vi "ArduinoCom.vi"(8 "error out":errorcluster, 10 "write buffer":string="b", 11 "VISA resource name out":refnum<visa-resource-name>) -> (0 "error out 2":errorcluster, 3 "VISA resource name out 2":refnum<visa-resource-name>)   [LabVIEW 2021]
panel:
  out "return count":u32=1
  out "Serial Settings:Number of Bytes at Serial Port":u32=3
  out "read buffer":string="a\r\n"
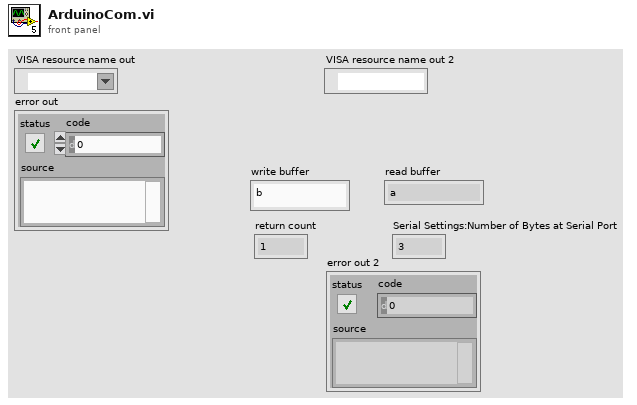
[diagram p1: front panel]
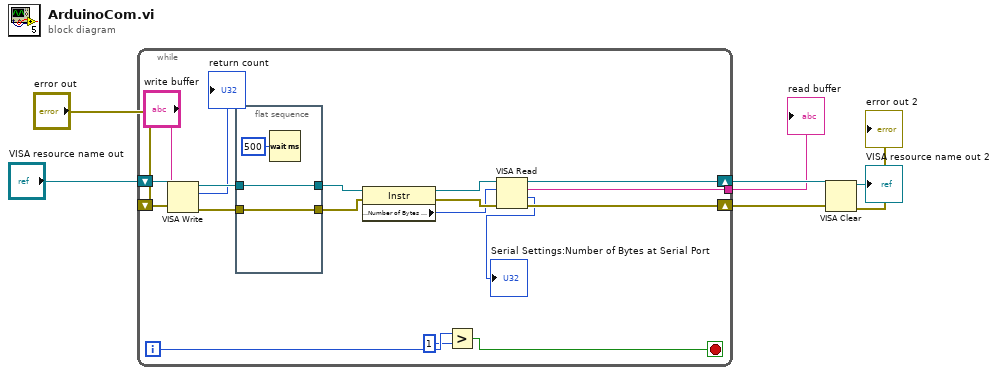
[diagram p0: block diagram]
diagram:
  n1 = while {
    tunnel: [w18] -> w5
    shift-right: [w19] -> w6
    shift-left: "error out" -> [w25]
    shift-right: [w20] -> w7
    shift-left: "VISA resource name out" -> [w24]
    i -> [w10]
    stop <- w8 stop-if-true
    n2 = VISA Write(VISA resource name=w24, write buffer="write buffer", error in (no error)=w25) -> (VISA resource name out=w22:refnum<visa-resource-name>, return count=→"return count":u32, error out=w21:errorcluster)
    n3 = flat-sequence {
      tunnel: w22 -> [w28]
      tunnel: [w28] -> w17
      tunnel: w21 -> [w27]
      tunnel: [w27] -> w16
      frame #0 {
        n4 = Wait (ms)(milliseconds to wait=u32 500) -> ()  [unwired: 1 out]
      }
    }
    n5 = property class="Instr"(reference=w17, error in=w16) -> (reference out=w15:refnum<visa-resource-name>, error out=w14:errorcluster, "Serial Settings:Number of Bytes at Serial Port"=w13:u32)
    n6 = Greater?(x=w10, y=1) -> (0:w8:bool)
    n7 = VISA Read(VISA resource name=w15, byte count=w13, error in (no error)=w14) -> (VISA resource name out=w20:refnum<visa-resource-name>, read buffer=w18:string, return count=→"Serial Settings:Number of Bytes at Serial Port":u32, error out=w19:errorcluster)
  }
  "read buffer" <- w5
  n8 = VISA Clear(VISA resource name=w7, error in (no error)=w6) -> (VISA resource name out=→"VISA resource name out 2":refnum<visa-resource-name>, error out=→"error out 2":errorcluster)
